vi "Actor Core.vi"(8 "error in (no error)":errorcluster, 11 "Mag Lab Measure Interface in":refnum<class "XY Plot.lvclass">) -> (0 "error out":errorcluster, 3 "Actor Framework.lvlib:Actor":refnum<class "Actor.lvclass">)   [LabVIEW 2019, in "XY Plot.lvclass"]
uses:
  XY Plot.lvclass
  C:/GitHub/LabActor/Template Module/Template Module.lvclass
  C:/Program Files/National Instruments/LabVIEW 2019/vi.lib/ActorFramework/Actor/Actor.lvclass
  <vilib>/ActorFramework/Actor/Actor.lvclass
  XY Plot.lvclass/XY Plot.ctl
  Template Module/Template Module.lvclass/Template Module.ctl
  <vilib>/ActorFramework/Actor/Actor.lvclass/Actor.ctl
  <vilib>/ActorFramework/Message Enqueuer/Message Enqueuer.lvclass/Message Enqueuer.ctl
  Controllers/Application Controller Messages/Plot Closed Msg/Plot Closed Msg.lvclass/Plot Closed Msg.ctl
  Plot Messages/Add file Msg/Add file Msg.lvclass/Add file Msg.ctl
  Template Module/Read stop event.vi
  <vilib>/ActorFramework/Message Enqueuer/Init from Existing Queue.vi
  <vilib>/ActorFramework/Message Enqueuer/Enqueue.vi
  <vilib>/ActorFramework/Stop Msg/Stop Msg.lvclass
  C:/Program Files/National Instruments/LabVIEW 2019/vi.lib/ActorFramework/Message/Message.lvclass
  Controllers/Application Controller Messages/Plot Closed Msg/Plot Closed Msg.lvclass
  Plot Messages/Add file Msg/Add file Msg.lvclass
  XY Plot Messages/Save keep old plots Msg/Save keep old plots Msg.lvclass
  Plot Messages/Replot Msg/Replot Msg.lvclass
  XY Plot Messages/Save defaults Msg/Save defaults Msg.lvclass
  <vilib>/ActorFramework/Message Priority Queue/Priority Enqueue.vi
  <vilib>/ActorFramework/Message Enqueuer/Message Enqueuer.lvclass
  Plot/Plot.lvclass
panel:
  in  "Set as default":bool
  in  "Keep old\nplots":bool
  in  "Open":bool
  in  "Exit":bool
  in  "Plots":cluster{"X":u16, "Y":u16}[](array[cluster]) {"Y" items=["Select channel...", "Time", "Y"]; "X" items=["Select channel...", "Time", "Y"]}
  out "XY Graph":cluster{dbl[], dbl[]}[](graph)
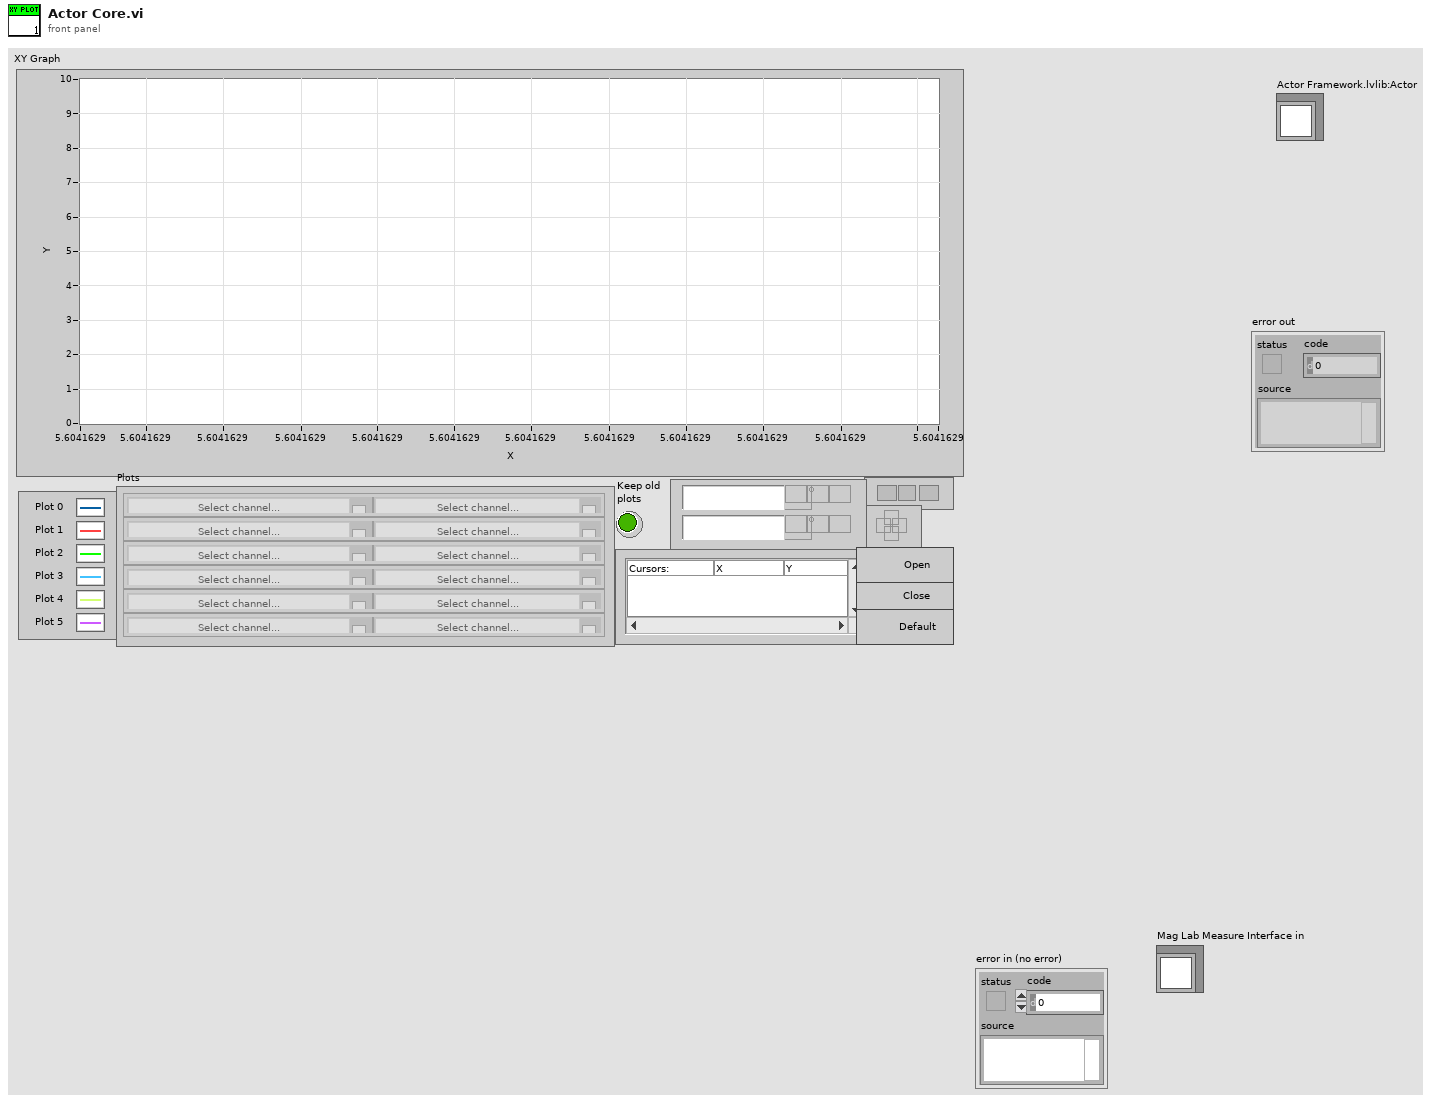
[diagram p1: front panel]
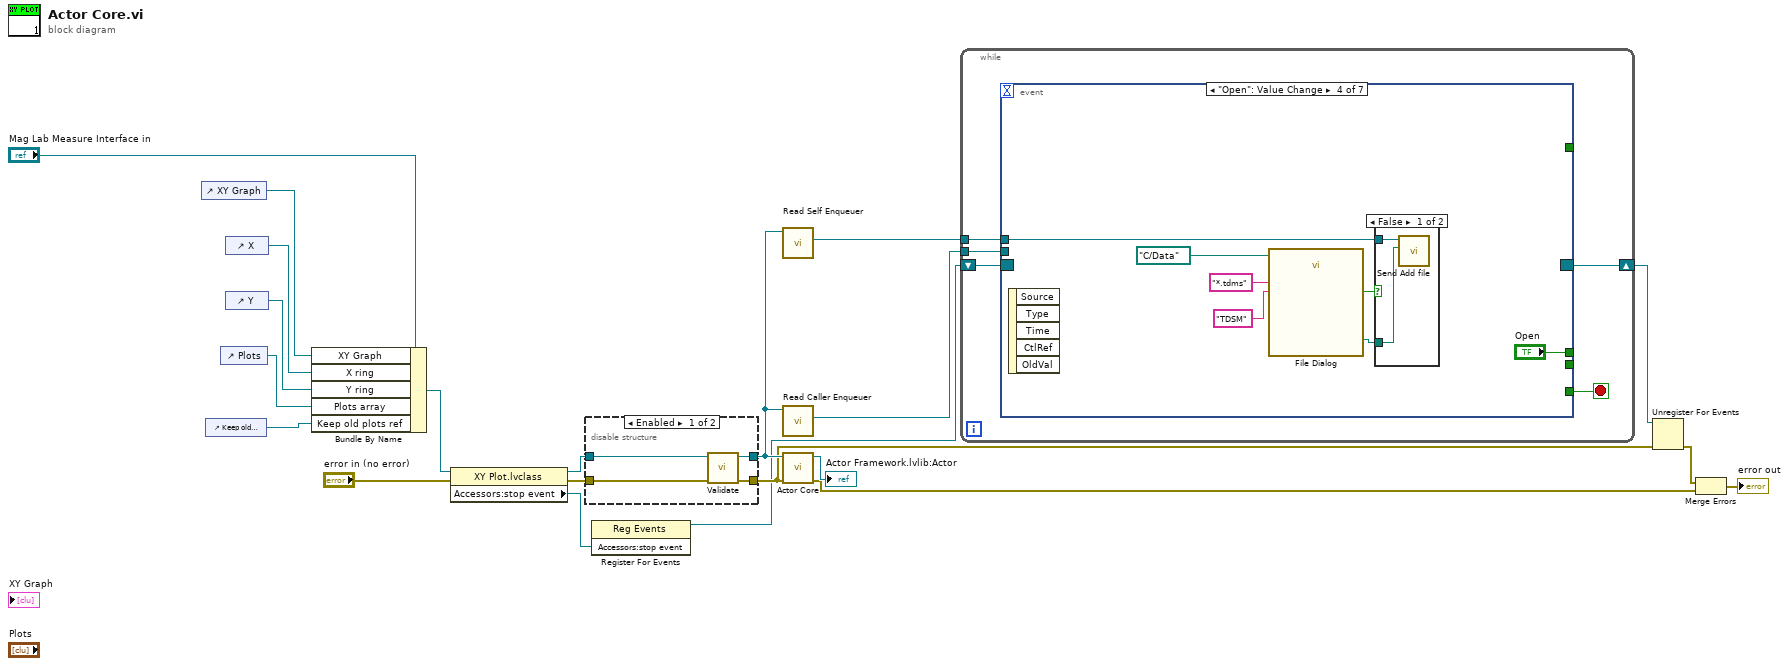
[diagram p0: block diagram]
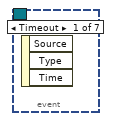
[diagram p2: hidden frame]
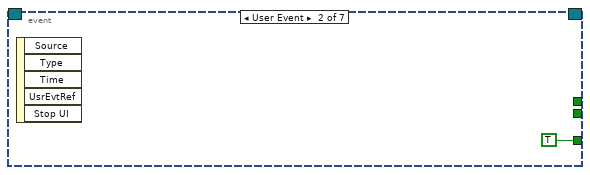
[diagram p3: hidden frame]
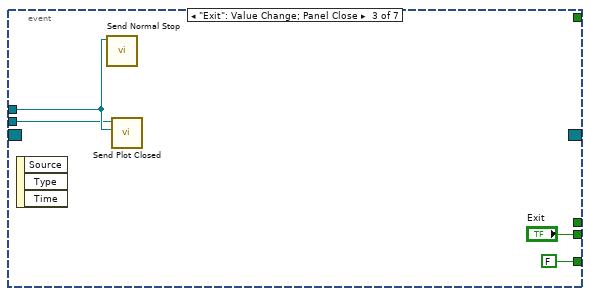
[diagram p4: hidden frame]
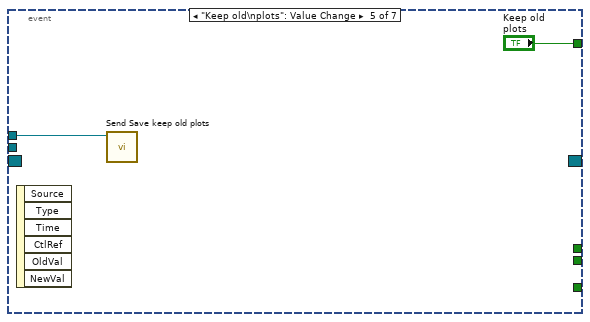
[diagram p6: hidden frame]
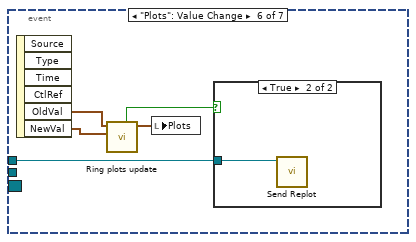
[diagram p7: hidden frame]
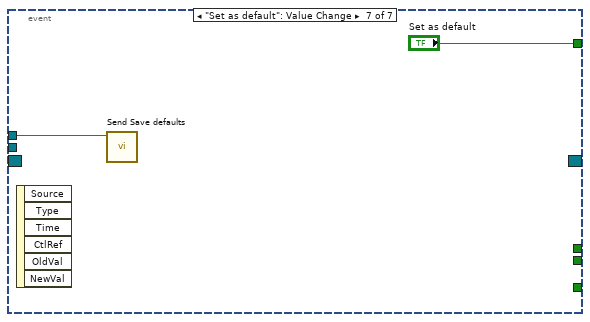
[diagram p9: hidden frame]
diagram:
  n1 = control-ref of="XY Graph"() -> (w14:refnum<vi>)
  n2 = control-ref of="Keep old\nplots"() -> (w11:refnum<vi>)
  n3 = control-ref of="Plots"() -> (w17:refnum<vi>)
  n4 = control-ref of="X"() -> (w16:refnum<vi>)
  n5 = control-ref of="Y"() -> (w15:refnum<vi>)
  n6 = Bundle By Name(cluster="Mag Lab Measure Interface in", "XY Graph"=w14, "X ring"=w16, "Y ring"=w15, "Plots array"=w17, "Keep old plots ref"=w11) -> (w7:refnum<class "XY Plot.lvclass">)
  n7 = property class="XY Plot.lvclass"(reference=w7, error in="error in (no error)") -> (reference out=w6:refnum<class "XY Plot.lvclass">, error out=w3:errorcluster, "Accessors:stop event"=w5:refnum<user-event>)
  n8 = disable-structure shown="Enabled" {
    disable-tunnel: [w25 w27] -> w10
    disable-tunnel: [w24 w26] -> w12
    disable-tunnel: w3 -> [w23 w27]
    disable-tunnel: w6 -> [w22 w26]
    frame Enabled {
      n9 = call-dynamic "Validate.vi"("error in (no error)"=w23, "MagLabGraph in"=w22) -> ("error out"=w25:errorcluster, "MagLabGraph out"=w24:refnum<class "XY Plot.lvclass">)  [unwired: 8 in]
    }
    frame Disabled {
    }
  }
  n10 = register-events(w5) -> (reference out=w2:refnum<event-registration>)  [unwired: 2 in, 1 out]
  n11 = call <vilib>:"Read Self Enqueuer.vi"("Actor"=w12) -> ("Self Enqueuer"=w19:refnum<class "Message Enqueuer.lvclass">)  [unwired: 10 in]
  n12 = call <vilib>:"Read Caller Enqueuer.vi"("Actor"=w12) -> ("Caller Enqueuer"=w13:refnum<class "Message Enqueuer.lvclass">)  [unwired: 10 in]
  n13 = call-parent "Actor Core.vi"("error in"=w10, "Measure Object in"=w12) -> ("error out"=w8:errorcluster, "Actor out"=→"Actor Framework.lvlib:Actor":refnum<class "Actor.lvclass">)  [unwired: 8 in]
  n14 = while {
    tunnel: w19 -> [w31]
    shift-right: [w29] -> w1
    shift-left: w2 -> [w32]
    tunnel: w13 -> [w28]
    stop <- w30 stop-if-true
    n15 = event shown="[3] \"Open\": Value Change" {
      selector: w32 -> [_ _ _ _ _ _ _]
      dyn-events: [_ _ _ _ _ _ _] -> w29
      timeout: _ -> [_ _ _ _ _ _ _]
      tunnel: w31 -> [_ _ w35 w39 w48 w49 w55]
      tunnel: [_ TRUE FALSE _ _ _ _] -> w30
      tunnel: [_ _ "Exit" _ _ _ _] -> _
      tunnel: [_ _ _ "Open" _ _ _] -> _
      tunnel: w28 -> [_ _ w34 _ _ _ _]
      tunnel: [_ _ _ _ "Keep old\nplots" _ "Set as default"] -> _
      event Timeout {
        n16 = event-data() -> ()  [unwired: 1 in, 3 out]
      }
      event User Event {
        n17 = event-data() -> ()  [unwired: 1 in, 5 out]
      }
      event "Exit": Value Change; Panel Close {
        n18 = event-data() -> ()  [unwired: 1 in, 3 out]
        n19 = call <vilib>:"Send Normal Stop.vi"("Message Enqueuer"=w35) -> ()  [unwired: 10 in, 1 out]
        n20 = call "Send Plot Closed.vi"("Closed plot"=w35, "Message Enqueuer"=w34) -> ()  [unwired: 8 in, 2 out]
      }
      event "Open": Value Change {
        n21 = event-data() -> ()  [unwired: 1 in, 5 out]
        n22 = call "File Dialog"("start path"=path "C:/Data", "pattern (all files)"="*.tdms", "pattern label"="TDSM") -> ("selected path"=w38:path, "cancelled"=w40:bool)  [unwired: 9 in, 2 out]
        n23 = case shown="False" w40 {
          tunnel: w39 -> [w46 _]
          tunnel: w38 -> [w45 _]
          frame False {
            n24 = call "Send Add file.vi"("File Path Control"=w45, "Message Enqueuer"=w46) -> ()  [unwired: 8 in, 2 out]
          }
          frame True {
          }
        }
      }
      event "Keep old\nplots": Value Change {
        n25 = event-data() -> ()  [unwired: 1 in, 6 out]
        n26 = call "Send Save keep old plots.vi"("Message Enqueuer"=w48) -> ()  [unwired: 9 in, 2 out]
      }
      event "Plots": Value Change {
        n27 = event-data() -> ("OldVal"=w51:cluster{"X":u16, "Y":u16}[], "NewVal"=w52:cluster{"X":u16, "Y":u16}[])  [unwired: 1 in, 4 out]
        n28 = call "Ring plots update.vi"("New Plots"=w52, "Old Plots"=w51) -> ("Plots"=w53:cluster{"X":u16, "Y":u16}[], "Replot?"=w50:bool)  [unwired: 8 in]
        n29 = local write "Plots"(w53) -> ()
        n30 = case shown="True" w50 {
          tunnel: w49 -> [_ w54]
          frame False {
          }
          frame True {
            n31 = call "Send Replot.vi"("Message Enqueuer"=w54) -> ()  [unwired: 9 in, 2 out]
          }
        }
      }
      event "Set as default": Value Change {
        n32 = event-data() -> ()  [unwired: 1 in, 6 out]
        n33 = call "Send Save defaults.vi"("Message Enqueuer"=w55) -> ()  [unwired: 9 in, 2 out]
      }
    }
  }
  n34 = Unregister For Events(event registration refnum=w1, error in=w10) -> (error out=w18:errorcluster)
  n35 = Merge Errors(w18, w8) -> (→"error out":errorcluster)
